vi "Test for reachability.vi"(8 "error in (no error)":errorcluster, 10 "must be directly reachable?":bool, 11 "address":refnum<class "Hostname Network Address.lvclass">) -> (0 "error out":errorcluster, 2 "found?":bool, 3 "address out":refnum<class "Generic Network Address.lvclass">)   [LabVIEW 2020, in "NI_WFCN.lvlib" / "Hostname Network Address.lvclass"]
doc: "Determine whether the specified address is reachable."
uses:
  <vilib>/net/WFCN/Addressing/Hostname Network Address/Hostname Network Address.lvclass
  e:/builds/penguin/labview/branches/2020/dev/dist/vi.lib/net/WFCN/Addressing/Generic Network Address/Generic Network Address.lvclass
  <vilib>/net/WFCN/Addressing/Generic Network Address/Generic Network Address.lvclass
  <vilib>/net/WFCN/Addressing/Hostname Network Address/Windows Scan DNS Config.vi
  <vilib>/net/WFCN/Addressing/Hostname Network Address/Windows run ipconfig.vi
  <vilib>/net/WFCN/Addressing/Hostname Network Address/Parse ipconfig.vi
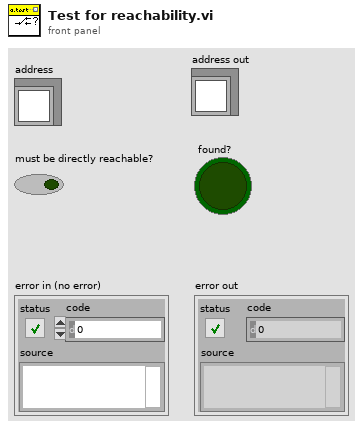
[diagram p1: front panel]
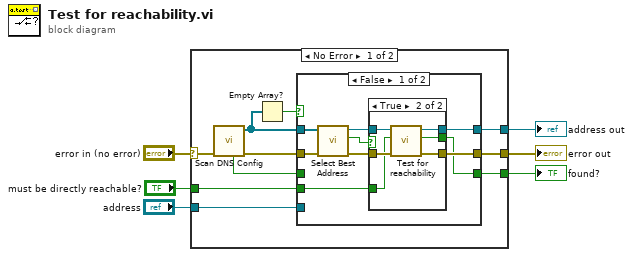
[diagram p0: block diagram]
diagram:
  n1 = case shown="No Error" "error in (no error)" {
    selector: "error in (no error)" -> [w11 w39]
    tunnel: [w14 w39] -> w4
    tunnel: "address" -> [w15 w38]
    tunnel: [w13 _] -> w3
    tunnel: [w12 w38] -> w2
    tunnel: "must be directly reachable?" -> [w7 _]
    frame No Error {
      n2 = call <vilib>:"Scan DNS Config.vi"("error in (no error)"=w11) -> ("error out"=w10:errorcluster, "DNS server addresses"=w9:refnum<class "Generic Network Address.lvclass">[], "found?"=w8:bool)  [unwired: 8 in]
      n3 = Empty Array?(array=w9) -> (empty?=w16:bool)
      n4 = case shown="False" w16 {
        tunnel: [w23 w37] -> w14
        tunnel: w10 -> [w22 w37]
        tunnel: w9 -> [w21 _]
        tunnel: w15 -> [_ w35]
        tunnel: w8 -> [_ w36]
        tunnel: [w18 w36] -> w13
        tunnel: [w19 w35] -> w12
        tunnel: w7 -> [w17 _]
        frame False {
          n5 = call <vilib>:"Select Best Address.vi"("error in (no error)"=w22, "addresses"=w21) -> ("error out"=w25:errorcluster, "found?"=w20:bool, "address"=w24:refnum<class "Generic Network Address.lvclass">)  [unwired: 7 in]
          n6 = case shown="True" w20 {
            selector: w20 -> [w26 _]
            tunnel: w24 -> [w27 w34]
            tunnel: w25 -> [w28 w33]
            tunnel: [w28 w31] -> w23
            tunnel: [w27 w32] -> w19
            tunnel: [w26 w30] -> w18
            tunnel: w17 -> [_ w29]
            frame False {
            }
            frame True {
              n7 = call-dynamic "Test for reachability.vi"("error in (no error)"=w33, "must be directly reachable?"=w29, "address"=w34) -> ("error out"=w31:errorcluster, "found?"=w30:bool, "address out"=w32:refnum<class "Generic Network Address.lvclass">)  [unwired: 6 in]
            }
          }
        }
        frame True {
        }
      }
    }
    frame Error {
    }
  }
  "error out" <- w4
  "found?" <- w3
  "address out" <- w2
